vi "ConfigureCamera.vi"() -> (0 "error out":errorcluster, 2 "New Image":T2, 3 "Refnum out":T1)   [LabVIEW 2024]
uses:
  <vilib>/vision/Image Controls.llb/IMAQ Image.ctl
  <vilib>/userDefined/High Color/IMAQdx.ctl
  <vilib>/Utility/error.llb/DialogType.ctl
  <vilib>/vision/driver/IMAQdx.llb/IMAQdx Camera Control Mode.ctl
  <vilib>/vision/driver/NI_Vision_Acquisition_Software.lvlib
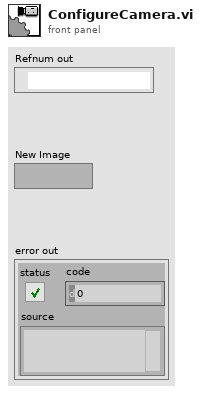
[diagram p1: front panel]
types:
  T1 = typedef "IMAQdx.ctl" = refnum<k21>
  T2 = typedef "IMAQ Image.ctl" = refnum<image>
  T3 = typedef "DialogType.ctl" = u16
  T4 = typedef "NI_Vision_Acquisition_Software.lvlib/IMAQdx Camera Control Mode.ctl" = enum32{"Controller", "Listener"}
  T5 = typedef "Image Type" = u32
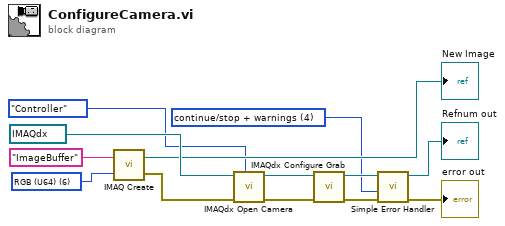
[diagram p0: block diagram]
diagram:
  w6 = T3 4 items=["no dialog", "OK message", "continue or stop message", "OK message + warnings", "continue/stop + warnings"] ("type of dialog (OK msg:1)")
  w4 = T5 6 items=["Grayscale (U8)", "Grayscale (I16)", "Grayscale (SGL)", "Complex (CSG)", "RGB (U32)", "HSL (U32)", "RGB (U64)", "Grayscale (U16)"] ("Image Type")
  n1 = call "IMAQ Create"("Image Name"="ImageBuffer", "Image Type"=w4) -> ("New Image"=→"New Image":T2, "error out"=w10:errorcluster)  [unwired: 3 in]
  n2 = call <vilib>:"IMAQdx Open Camera.vi"("Camera Control Mode"=IMAQdx_Camera_Control_Mode."Controller", "error in"=w10, "Session In"=T1 "cam0" ("Refnum in")) -> ("error out"=w2:errorcluster, "Session Out"=w1:T1)  [unwired: 7 in]
  n3 = call <vilib>:"IMAQdx Configure Grab.vi"("error in"=w2, "Session In"=w1) -> ("error out"=w11:errorcluster, "Session Out"=→"Refnum out":T1)  [unwired: 8 in]
  n4 = call <vilib>:"Simple Error Handler.vi"("type of dialog (OK msg:1)"=w6, "error in (no error)"=w11) -> ("error out"=→"error out":errorcluster)  [unwired: 3 in, 4 out]
